vi "CAN_initialize3.vi"() -> (0 "Array 2":errorcluster[](array[cluster]), 1 "Array":refnum<class "sbCANopenBaseClass.lvclass">[](array[class]), 2 "Motor order":i32[](array[numeric])=[3, 6, 9, 12, 2, 7, 8, 13, 4, 5, 10, 11, 1, 14])   [LabVIEW 2024]
uses:
  <vilib>/addons/Maxon Motor/EPOS2 CANopen/CANopen/sbCANopenBaseClass.lvclass
  <vilib>/addons/Maxon Motor/EPOS2 CANopen/EPOS2 Support Files/Typedefs/EPOS2 Config Data Input Current.ctl
  <vilib>/addons/Maxon Motor/EPOS2 CANopen/EPOS2 Support Files/Typedefs/EPOS2 Velocity Units.ctl
  <vilib>/addons/Maxon Motor/EPOS2 CANopen/EPOS2 Support Files/Polymorphic SubVIs/Config/EPOS2 Current Mode Configure.vi
  <vilib>/addons/Maxon Motor/EPOS2 CANopen/EPOS2 Library.lvlib
  <vilib>/addons/Maxon Motor/EPOS2 CANopen/CANopen/CANopen IndCom Interface/sdCANopenIndCom.lvclass
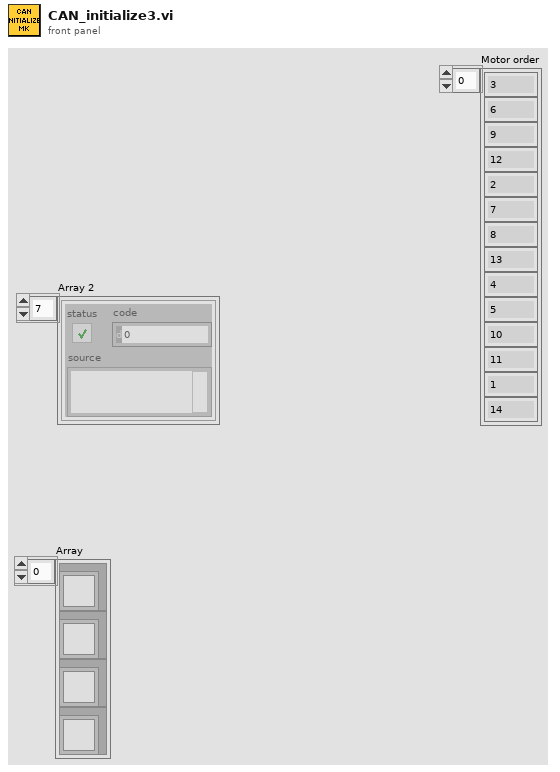
[diagram p1: front panel]
types:
  T1 = typedef "EPOS2 Library.lvlib/EPOS2 Config Data Input Current.ctl" = cluster{"Velocity Units":T2, "Max Velocity":i32}
  T2 = typedef "EPOS2 Library.lvlib/EPOS2 Velocity Units.ctl" = i8
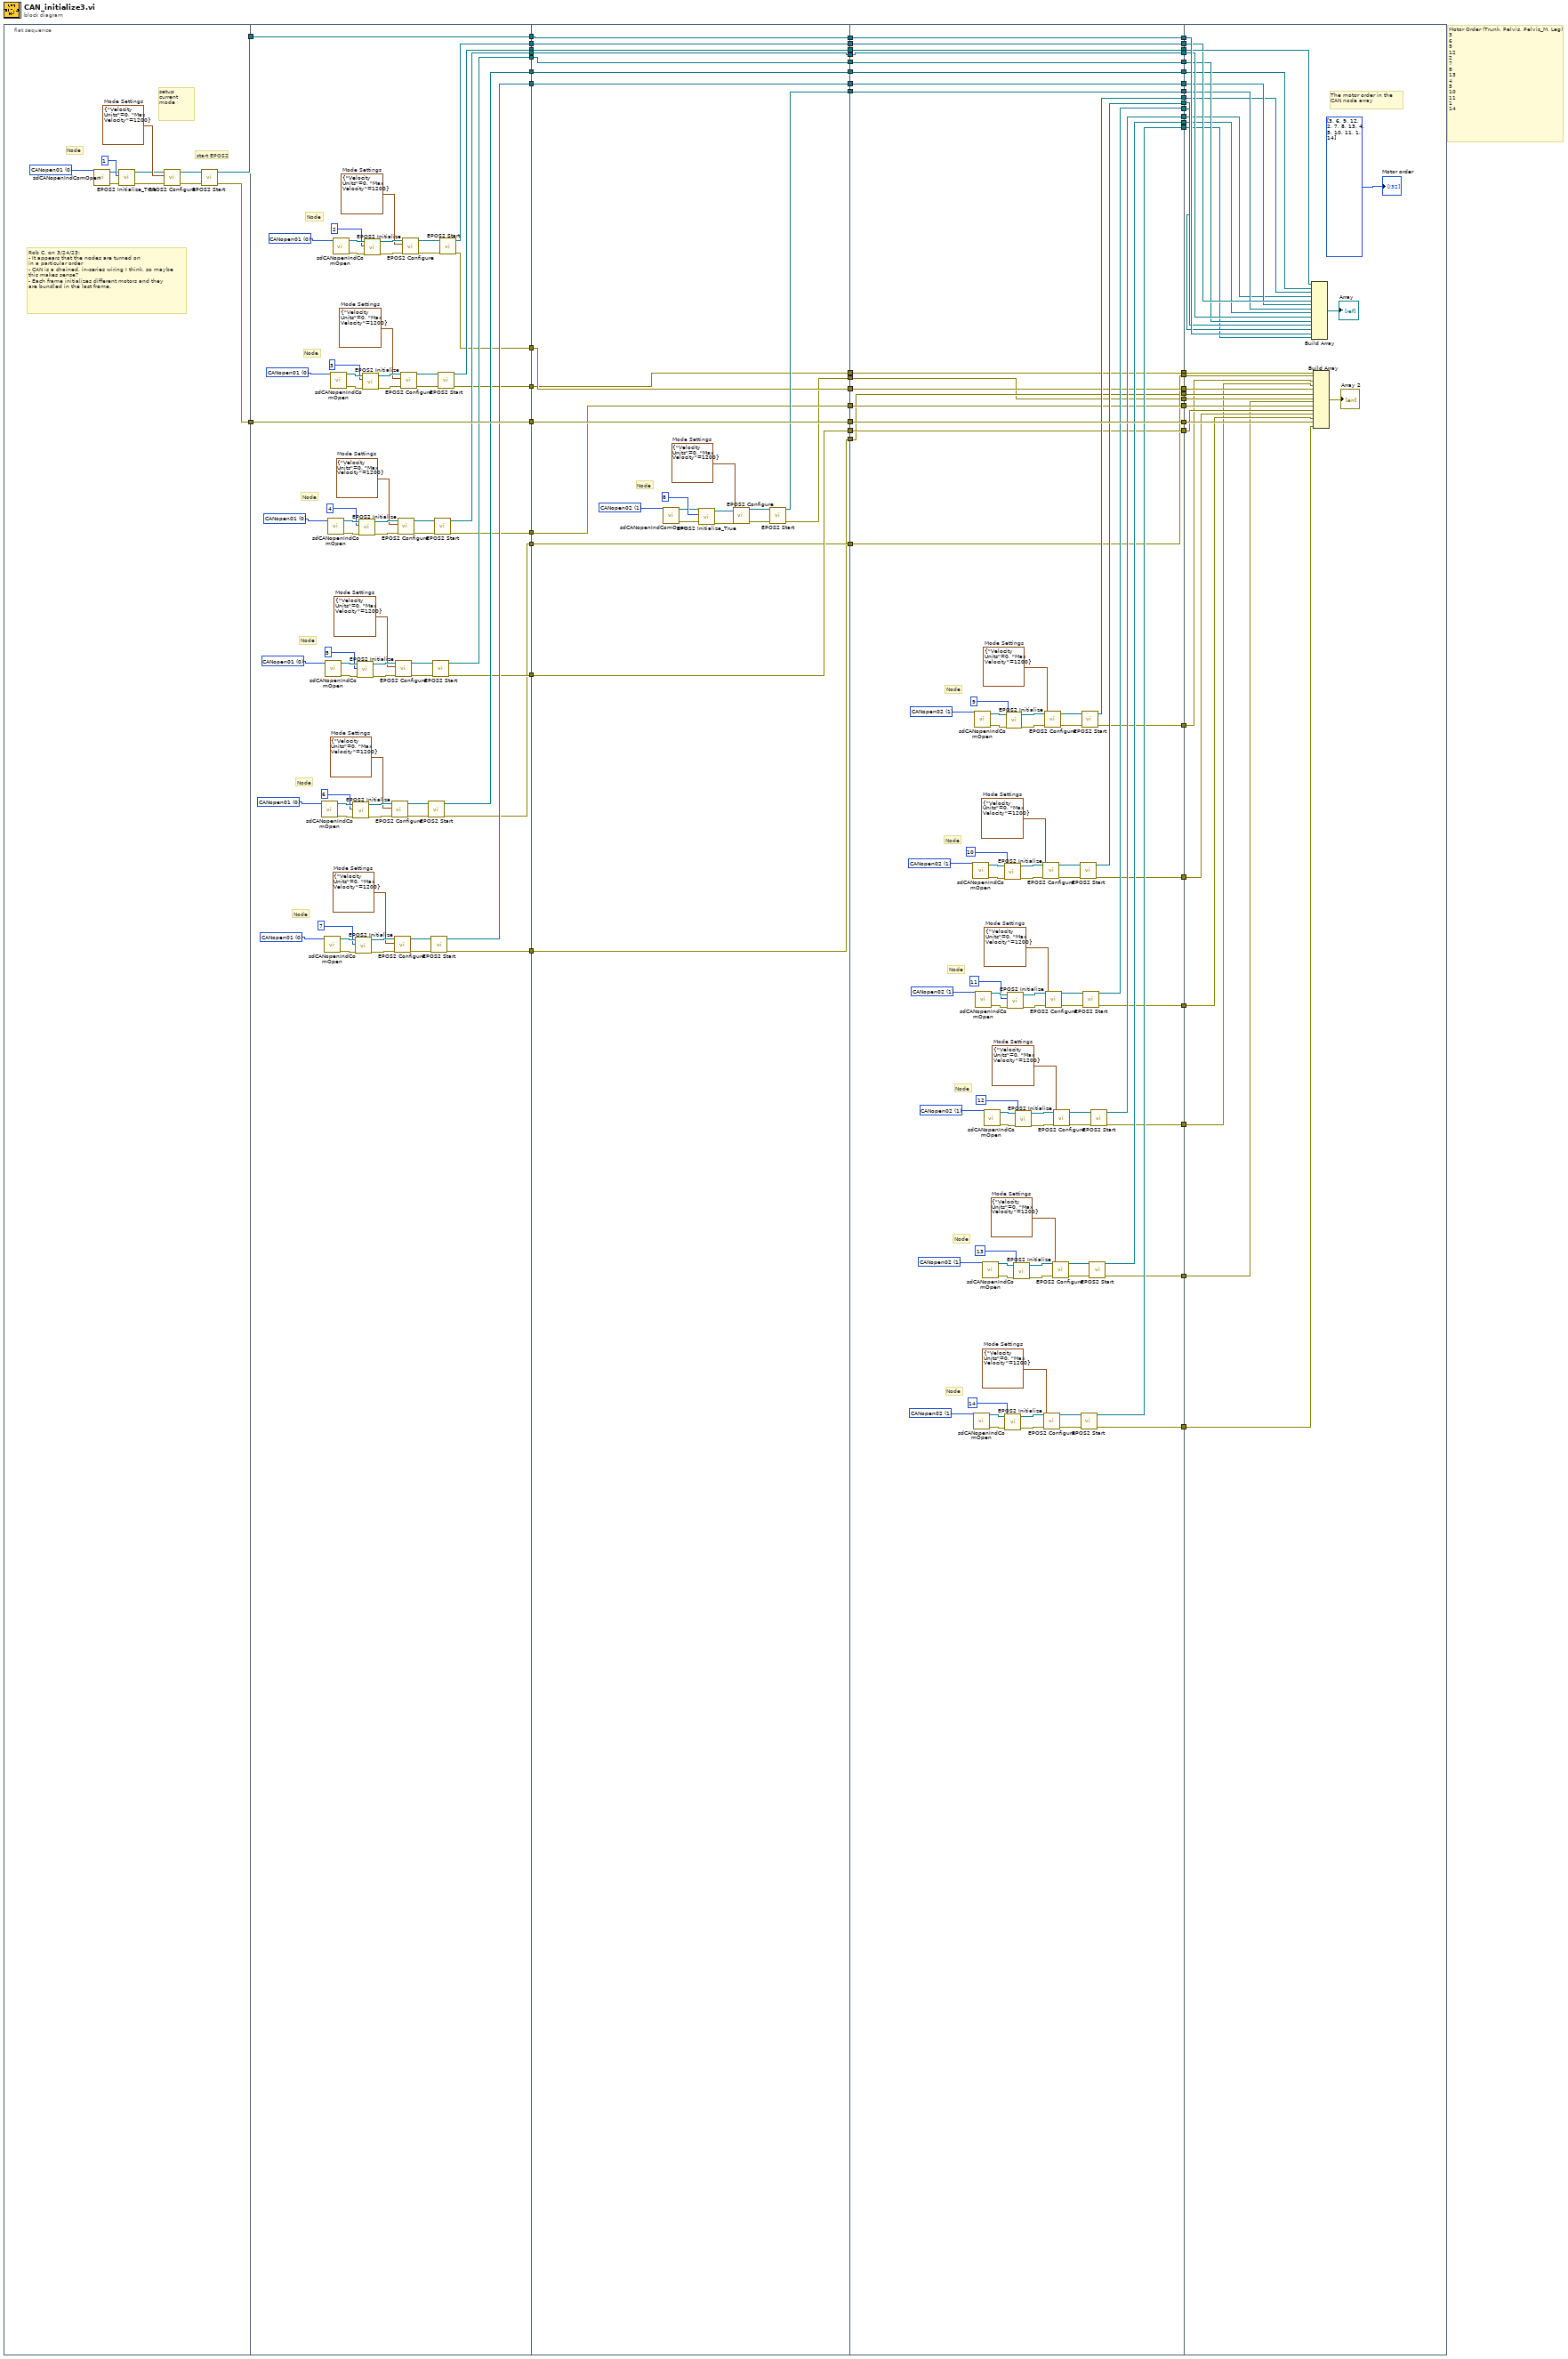
[diagram p0: block diagram]
diagram:
  # "Motor Order (Trunk, Pelvis, Pelvis_M, Leg)\n3\n6\n9\n12\n2\n7\n8\n13\n4\n5\n10\n11\n1\n14"
  n1 = flat-sequence {
    tunnel: [w62] -> w60
    tunnel: [w61] -> w56
    tunnel: w60 -> [w85]
    tunnel: [w85] -> w57
    tunnel: w56 -> [w84]
    tunnel: [w84] -> w53
    tunnel: [w83] -> w50
    tunnel: [w82] -> w49
    tunnel: [w81] -> w46
    tunnel: [w80] -> w43
    tunnel: [w79] -> w38
    tunnel: [w78] -> w35
    tunnel: [w77] -> w26
    tunnel: [w76] -> w21
    tunnel: [w75] -> w18
    tunnel: [w74] -> w15
    tunnel: [w73] -> w14
    tunnel: [w72] -> w10
    tunnel: [w155] -> w58
    tunnel: w57 -> [w155]
    tunnel: [w154] -> w54
    tunnel: w53 -> [w154]
    tunnel: [w153] -> w51
    tunnel: w50 -> [w153]
    tunnel: w49 -> [w152]
    tunnel: [w152] -> w47
    tunnel: w46 -> [w151]
    tunnel: [w151] -> w44
    tunnel: w43 -> [w150]
    tunnel: [w150] -> w41
    tunnel: [w149] -> w39
    tunnel: w38 -> [w149]
    tunnel: [w148] -> w36
    tunnel: w35 -> [w148]
    tunnel: [w147] -> w34
    tunnel: w26 -> [w146]
    tunnel: [w146] -> w24
    tunnel: [w145] -> w22
    tunnel: w21 -> [w145]
    tunnel: [w144] -> w19
    tunnel: w18 -> [w144]
    tunnel: [w143] -> w16
    tunnel: w15 -> [w143]
    tunnel: w14 -> [w142]
    tunnel: [w142] -> w12
    tunnel: [w141] -> w11
    tunnel: w10 -> [w141]
    tunnel: [w140] -> w8
    tunnel: [w192] -> w59
    tunnel: w58 -> [w192]
    tunnel: [w191] -> w55
    tunnel: w54 -> [w191]
    tunnel: [w190] -> w52
    tunnel: w51 -> [w190]
    tunnel: [w189] -> w48
    tunnel: w47 -> [w189]
    tunnel: [w188] -> w45
    tunnel: w44 -> [w188]
    tunnel: [w187] -> w42
    tunnel: w41 -> [w187]
    tunnel: [w186] -> w40
    tunnel: w39 -> [w186]
    tunnel: [w185] -> w37
    tunnel: w36 -> [w185]
    tunnel: w34 -> [w184]
    tunnel: [w184] -> w33
    tunnel: [w183] -> w32
    tunnel: [w182] -> w31
    tunnel: [w181] -> w30
    tunnel: [w180] -> w29
    tunnel: [w179] -> w28
    tunnel: [w178] -> w27
    tunnel: [w177] -> w25
    tunnel: w24 -> [w177]
    tunnel: [w176] -> w23
    tunnel: w22 -> [w176]
    tunnel: [w175] -> w20
    tunnel: w19 -> [w175]
    tunnel: [w174] -> w17
    tunnel: w16 -> [w174]
    tunnel: [w173] -> w13
    tunnel: w12 -> [w173]
    tunnel: w11 -> [w172]
    tunnel: [w172] -> w9
    tunnel: w8 -> [w171]
    tunnel: [w171] -> w7
    tunnel: [w170] -> w6
    tunnel: [w169] -> w5
    tunnel: [w168] -> w4
    tunnel: [w167] -> w3
    tunnel: [w166] -> w2
    tunnel: [w165] -> w1
    tunnel: w59 -> [w277]
    tunnel: w55 -> [w276]
    tunnel: w52 -> [w272]
    tunnel: w48 -> [w273]
    tunnel: w45 -> [w271]
    tunnel: w42 -> [w270]
    tunnel: w40 -> [w269]
    tunnel: w37 -> [w268]
    tunnel: w33 -> [w267]
    tunnel: w32 -> [w266]
    tunnel: w31 -> [w265]
    tunnel: w30 -> [w264]
    tunnel: w29 -> [w263]
    tunnel: w28 -> [w262]
    tunnel: w27 -> [w261]
    tunnel: w25 -> [w260]
    tunnel: w23 -> [w259]
    tunnel: w20 -> [w258]
    tunnel: w17 -> [w257]
    tunnel: w13 -> [w256]
    tunnel: w9 -> [w255]
    tunnel: w7 -> [w254]
    tunnel: w6 -> [w253]
    tunnel: w5 -> [w252]
    tunnel: w4 -> [w251]
    tunnel: w3 -> [w250]
    tunnel: w2 -> [w249]
    tunnel: w1 -> [w248]
    frame #0 {
      w70 = u32 0 items=["CANopen01", "CANopen02", "CANopen03", "CANopen04", "CANopen05", "CANopen06", "CANopen07", "CANopen08", "CANopen09", "CANopen10", "CANopen11", "CANopen12", "CANopen13", "CANopen14", "CANopen15", "CANopen16", "CANopen17", "CANopen18", "CANopen19", "CANopen20", "CANopen21", "CANopen22", "CANopen23", "CANopen24", "CANopen25", "CANopen26", "CANopen27", "CANopen28", "CANopen29", "CANopen30", "CANopen31", "CANopen32"] ("Interface Name")
      w71 = T1 {"Velocity Units"=0, "Max Velocity"=1200}  # Mode Settings
      # "Rob C. on 3/24/23:\n- It appears that the nodes are turned on\nin a particular order\n- CAN is a chained, in-series wiring I think, so maybe\nthis makes sense? \n- Each frame initializes different motors and they \nare bundled in the last frame."
      # "Node"
      # "start EPOS2"
      # "setup current mode"
      n2 = call <vilib>:"sdCANopenIndComOpen.vi"("Interface Name"=w70) -> ("error out"=w67:errorcluster, "SD CANopen Comm out"=w63:refnum<class "sbCANopenBaseClass.lvclass">)  [unwired: 9 in]
      n3 = call <vilib>:"EPOS2 Initialize_True.vi"("error in"=w67, "Node ID"=u8 1, "CAN Session In"=w63) -> ("error out"=w68:errorcluster, "CANopen Session Out"=w65:refnum<class "sbCANopenBaseClass.lvclass">)  [unwired: 7 in]
      n4 = call-poly <vilib>:"EPOS2 Configure.vi"("error in"=w68, "Mode Settings"=w71, "CANopen Session In"=w65) -> ("error out"=w66:errorcluster, "CANopen Session Out"=w64:refnum<class "sbCANopenBaseClass.lvclass">)  [unwired: 7 in]
      n5 = call <vilib>:"EPOS2 Start.vi"("error in"=w66, "CANopen Session In"=w64) -> ("error out"=w61:errorcluster, "CANopen Session Out"=w62:refnum<class "sbCANopenBaseClass.lvclass">)  [unwired: 8 in]
    }
    frame #1 {
      w89 = u32 0 items=["CANopen01", "CANopen02", "CANopen03", "CANopen04", "CANopen05", "CANopen06", "CANopen07", "CANopen08", "CANopen09", "CANopen10", "CANopen11", "CANopen12", "CANopen13", "CANopen14", "CANopen15", "CANopen16", "CANopen17", "CANopen18", "CANopen19", "CANopen20", "CANopen21", "CANopen22", "CANopen23", "CANopen24", "CANopen25", "CANopen26", "CANopen27", "CANopen28", "CANopen29", "CANopen30", "CANopen31", "CANopen32"] ("Interface Name")
      w90 = T1 {"Velocity Units"=0, "Max Velocity"=1200}  # Mode Settings
      w97 = u32 0 items=["CANopen01", "CANopen02", "CANopen03", "CANopen04", "CANopen05", "CANopen06", "CANopen07", "CANopen08", "CANopen09", "CANopen10", "CANopen11", "CANopen12", "CANopen13", "CANopen14", "CANopen15", "CANopen16", "CANopen17", "CANopen18", "CANopen19", "CANopen20", "CANopen21", "CANopen22", "CANopen23", "CANopen24", "CANopen25", "CANopen26", "CANopen27", "CANopen28", "CANopen29", "CANopen30", "CANopen31", "CANopen32"] ("Interface Name")
      w98 = T1 {"Velocity Units"=0, "Max Velocity"=1200}  # Mode Settings
      w109 = u32 0 items=["CANopen01", "CANopen02", "CANopen03", "CANopen04", "CANopen05", "CANopen06", "CANopen07", "CANopen08", "CANopen09", "CANopen10", "CANopen11", "CANopen12", "CANopen13", "CANopen14", "CANopen15", "CANopen16", "CANopen17", "CANopen18", "CANopen19", "CANopen20", "CANopen21", "CANopen22", "CANopen23", "CANopen24", "CANopen25", "CANopen26", "CANopen27", "CANopen28", "CANopen29", "CANopen30", "CANopen31", "CANopen32"] ("Interface Name")
      w110 = T1 {"Velocity Units"=0, "Max Velocity"=1200}  # Mode Settings
      w117 = u32 0 items=["CANopen01", "CANopen02", "CANopen03", "CANopen04", "CANopen05", "CANopen06", "CANopen07", "CANopen08", "CANopen09", "CANopen10", "CANopen11", "CANopen12", "CANopen13", "CANopen14", "CANopen15", "CANopen16", "CANopen17", "CANopen18", "CANopen19", "CANopen20", "CANopen21", "CANopen22", "CANopen23", "CANopen24", "CANopen25", "CANopen26", "CANopen27", "CANopen28", "CANopen29", "CANopen30", "CANopen31", "CANopen32"] ("Interface Name")
      w118 = T1 {"Velocity Units"=0, "Max Velocity"=1200}  # Mode Settings
      w125 = u32 0 items=["CANopen01", "CANopen02", "CANopen03", "CANopen04", "CANopen05", "CANopen06", "CANopen07", "CANopen08", "CANopen09", "CANopen10", "CANopen11", "CANopen12", "CANopen13", "CANopen14", "CANopen15", "CANopen16", "CANopen17", "CANopen18", "CANopen19", "CANopen20", "CANopen21", "CANopen22", "CANopen23", "CANopen24", "CANopen25", "CANopen26", "CANopen27", "CANopen28", "CANopen29", "CANopen30", "CANopen31", "CANopen32"] ("Interface Name")
      w126 = T1 {"Velocity Units"=0, "Max Velocity"=1200}  # Mode Settings
      w133 = u32 0 items=["CANopen01", "CANopen02", "CANopen03", "CANopen04", "CANopen05", "CANopen06", "CANopen07", "CANopen08", "CANopen09", "CANopen10", "CANopen11", "CANopen12", "CANopen13", "CANopen14", "CANopen15", "CANopen16", "CANopen17", "CANopen18", "CANopen19", "CANopen20", "CANopen21", "CANopen22", "CANopen23", "CANopen24", "CANopen25", "CANopen26", "CANopen27", "CANopen28", "CANopen29", "CANopen30", "CANopen31", "CANopen32"] ("Interface Name")
      w134 = T1 {"Velocity Units"=0, "Max Velocity"=1200}  # Mode Settings
      # "Node"
      # "Node"
      # "Node"
      # "Node"
      # "Node"
      # "Node"
      n6 = call <vilib>:"sdCANopenIndComOpen.vi"("Interface Name"=w97) -> ("error out"=w102:errorcluster, "SD CANopen Comm out"=w96:refnum<class "sbCANopenBaseClass.lvclass">)  [unwired: 9 in]
      n7 = call <vilib>:"sdCANopenIndComOpen.vi"("Interface Name"=w89) -> ("error out"=w94:errorcluster, "SD CANopen Comm out"=w88:refnum<class "sbCANopenBaseClass.lvclass">)  [unwired: 9 in]
      n8 = call <vilib>:"sdCANopenIndComOpen.vi"("Interface Name"=w109) -> ("error out"=w114:errorcluster, "SD CANopen Comm out"=w108:refnum<class "sbCANopenBaseClass.lvclass">)  [unwired: 9 in]
      n9 = call <vilib>:"sdCANopenIndComOpen.vi"("Interface Name"=w117) -> ("error out"=w122:errorcluster, "SD CANopen Comm out"=w116:refnum<class "sbCANopenBaseClass.lvclass">)  [unwired: 9 in]
      n10 = call <vilib>:"sdCANopenIndComOpen.vi"("Interface Name"=w125) -> ("error out"=w130:errorcluster, "SD CANopen Comm out"=w124:refnum<class "sbCANopenBaseClass.lvclass">)  [unwired: 9 in]
      n11 = call <vilib>:"sdCANopenIndComOpen.vi"("Interface Name"=w133) -> ("error out"=w138:errorcluster, "SD CANopen Comm out"=w132:refnum<class "sbCANopenBaseClass.lvclass">)  [unwired: 9 in]
      n12 = call <vilib>:"EPOS2 Initialize.vi"("error in"=w102, "Node ID"=u8 6, "CAN Session In"=w96) -> ("error out"=w103:errorcluster, "CANopen Session Out"=w100:refnum<class "sbCANopenBaseClass.lvclass">)  [unwired: 1 in, 6 out]
      n13 = call <vilib>:"EPOS2 Initialize.vi"("error in"=w94, "Node ID"=u8 7, "CAN Session In"=w88) -> ("error out"=w95:errorcluster, "CANopen Session Out"=w92:refnum<class "sbCANopenBaseClass.lvclass">)  [unwired: 1 in, 6 out]
      n14 = call <vilib>:"EPOS2 Initialize.vi"("error in"=w114, "Node ID"=u8 5, "CAN Session In"=w108) -> ("error out"=w115:errorcluster, "CANopen Session Out"=w112:refnum<class "sbCANopenBaseClass.lvclass">)  [unwired: 1 in, 6 out]
      n15 = call <vilib>:"EPOS2 Initialize.vi"("error in"=w122, "Node ID"=u8 4, "CAN Session In"=w116) -> ("error out"=w123:errorcluster, "CANopen Session Out"=w120:refnum<class "sbCANopenBaseClass.lvclass">)  [unwired: 1 in, 6 out]
      n16 = call <vilib>:"EPOS2 Initialize.vi"("error in"=w130, "Node ID"=u8 3, "CAN Session In"=w124) -> ("error out"=w131:errorcluster, "CANopen Session Out"=w128:refnum<class "sbCANopenBaseClass.lvclass">)  [unwired: 1 in, 6 out]
      n17 = call <vilib>:"EPOS2 Initialize.vi"("error in"=w138, "Node ID"=u8 2, "CAN Session In"=w132) -> ("error out"=w139:errorcluster, "CANopen Session Out"=w136:refnum<class "sbCANopenBaseClass.lvclass">)  [unwired: 1 in, 6 out]
      n18 = call-poly <vilib>:"EPOS2 Configure.vi"("error in"=w103, "Mode Settings"=w98, "CANopen Session In"=w100) -> ("error out"=w101:errorcluster, "CANopen Session Out"=w99:refnum<class "sbCANopenBaseClass.lvclass">)  [unwired: 7 in]
      n19 = call-poly <vilib>:"EPOS2 Configure.vi"("error in"=w95, "Mode Settings"=w90, "CANopen Session In"=w92) -> ("error out"=w93:errorcluster, "CANopen Session Out"=w91:refnum<class "sbCANopenBaseClass.lvclass">)  [unwired: 7 in]
      n20 = call-poly <vilib>:"EPOS2 Configure.vi"("error in"=w115, "Mode Settings"=w110, "CANopen Session In"=w112) -> ("error out"=w113:errorcluster, "CANopen Session Out"=w111:refnum<class "sbCANopenBaseClass.lvclass">)  [unwired: 7 in]
      n21 = call-poly <vilib>:"EPOS2 Configure.vi"("error in"=w123, "Mode Settings"=w118, "CANopen Session In"=w120) -> ("error out"=w121:errorcluster, "CANopen Session Out"=w119:refnum<class "sbCANopenBaseClass.lvclass">)  [unwired: 7 in]
      n22 = call-poly <vilib>:"EPOS2 Configure.vi"("error in"=w131, "Mode Settings"=w126, "CANopen Session In"=w128) -> ("error out"=w129:errorcluster, "CANopen Session Out"=w127:refnum<class "sbCANopenBaseClass.lvclass">)  [unwired: 7 in]
      n23 = call-poly <vilib>:"EPOS2 Configure.vi"("error in"=w139, "Mode Settings"=w134, "CANopen Session In"=w136) -> ("error out"=w137:errorcluster, "CANopen Session Out"=w135:refnum<class "sbCANopenBaseClass.lvclass">)  [unwired: 7 in]
      n24 = call <vilib>:"EPOS2 Start.vi"("error in"=w101, "CANopen Session In"=w99) -> ("error out"=w73:errorcluster, "CANopen Session Out"=w79:refnum<class "sbCANopenBaseClass.lvclass">)  [unwired: 8 in]
      n25 = call <vilib>:"EPOS2 Start.vi"("error in"=w93, "CANopen Session In"=w91) -> ("error out"=w72:errorcluster, "CANopen Session Out"=w78:refnum<class "sbCANopenBaseClass.lvclass">)  [unwired: 8 in]
      n26 = call <vilib>:"EPOS2 Start.vi"("error in"=w113, "CANopen Session In"=w111) -> ("error out"=w74:errorcluster, "CANopen Session Out"=w80:refnum<class "sbCANopenBaseClass.lvclass">)  [unwired: 8 in]
      n27 = call <vilib>:"EPOS2 Start.vi"("error in"=w121, "CANopen Session In"=w119) -> ("error out"=w75:errorcluster, "CANopen Session Out"=w81:refnum<class "sbCANopenBaseClass.lvclass">)  [unwired: 8 in]
      n28 = call <vilib>:"EPOS2 Start.vi"("error in"=w129, "CANopen Session In"=w127) -> ("error out"=w76:errorcluster, "CANopen Session Out"=w82:refnum<class "sbCANopenBaseClass.lvclass">)  [unwired: 8 in]
      n29 = call <vilib>:"EPOS2 Start.vi"("error in"=w137, "CANopen Session In"=w135) -> ("error out"=w77:errorcluster, "CANopen Session Out"=w83:refnum<class "sbCANopenBaseClass.lvclass">)  [unwired: 8 in]
    }
    frame #2 {
      w162 = u32 1 items=["CANopen01", "CANopen02", "CANopen03", "CANopen04", "CANopen05", "CANopen06", "CANopen07", "CANopen08", "CANopen09", "CANopen10", "CANopen11", "CANopen12", "CANopen13", "CANopen14", "CANopen15", "CANopen16", "CANopen17", "CANopen18", "CANopen19", "CANopen20", "CANopen21", "CANopen22", "CANopen23", "CANopen24", "CANopen25", "CANopen26", "CANopen27", "CANopen28", "CANopen29", "CANopen30", "CANopen31", "CANopen32"] ("Interface Name")
      w161 = T1 {"Velocity Units"=0, "Max Velocity"=1200}  # Mode Settings
      # "Node"
      n30 = call <vilib>:"sdCANopenIndComOpen.vi"("Interface Name"=w162) -> ("error out"=w157:errorcluster, "SD CANopen Comm out"=w159:refnum<class "sbCANopenBaseClass.lvclass">)  [unwired: 9 in]
      n31 = call <vilib>:"EPOS2 Initialize_True.vi"("error in"=w157, "Node ID"=u8 8, "CAN Session In"=w159) -> ("error out"=w156:errorcluster, "CANopen Session Out"=w158:refnum<class "sbCANopenBaseClass.lvclass">)  [unwired: 7 in]
      n32 = call-poly <vilib>:"EPOS2 Configure.vi"("error in"=w156, "Mode Settings"=w161, "CANopen Session In"=w158) -> ("error out"=w163:errorcluster, "CANopen Session Out"=w164:refnum<class "sbCANopenBaseClass.lvclass">)  [unwired: 7 in]
      n33 = call <vilib>:"EPOS2 Start.vi"("error in"=w163, "CANopen Session In"=w164) -> ("error out"=w140:errorcluster, "CANopen Session Out"=w147:refnum<class "sbCANopenBaseClass.lvclass">)  [unwired: 8 in]
    }
    frame #3 {
      w201 = u32 1 items=["CANopen01", "CANopen02", "CANopen03", "CANopen04", "CANopen05", "CANopen06", "CANopen07", "CANopen08", "CANopen09", "CANopen10", "CANopen11", "CANopen12", "CANopen13", "CANopen14", "CANopen15", "CANopen16", "CANopen17", "CANopen18", "CANopen19", "CANopen20", "CANopen21", "CANopen22", "CANopen23", "CANopen24", "CANopen25", "CANopen26", "CANopen27", "CANopen28", "CANopen29", "CANopen30", "CANopen31", "CANopen32"] ("Interface Name")
      w200 = T1 {"Velocity Units"=0, "Max Velocity"=1200}  # Mode Settings
      w198 = u32 1 items=["CANopen01", "CANopen02", "CANopen03", "CANopen04", "CANopen05", "CANopen06", "CANopen07", "CANopen08", "CANopen09", "CANopen10", "CANopen11", "CANopen12", "CANopen13", "CANopen14", "CANopen15", "CANopen16", "CANopen17", "CANopen18", "CANopen19", "CANopen20", "CANopen21", "CANopen22", "CANopen23", "CANopen24", "CANopen25", "CANopen26", "CANopen27", "CANopen28", "CANopen29", "CANopen30", "CANopen31", "CANopen32"] ("Interface Name")
      w197 = T1 {"Velocity Units"=0, "Max Velocity"=1200}  # Mode Settings
      w195 = u32 1 items=["CANopen01", "CANopen02", "CANopen03", "CANopen04", "CANopen05", "CANopen06", "CANopen07", "CANopen08", "CANopen09", "CANopen10", "CANopen11", "CANopen12", "CANopen13", "CANopen14", "CANopen15", "CANopen16", "CANopen17", "CANopen18", "CANopen19", "CANopen20", "CANopen21", "CANopen22", "CANopen23", "CANopen24", "CANopen25", "CANopen26", "CANopen27", "CANopen28", "CANopen29", "CANopen30", "CANopen31", "CANopen32"] ("Interface Name")
      w194 = T1 {"Velocity Units"=0, "Max Velocity"=1200}  # Mode Settings
      w228 = u32 1 items=["CANopen01", "CANopen02", "CANopen03", "CANopen04", "CANopen05", "CANopen06", "CANopen07", "CANopen08", "CANopen09", "CANopen10", "CANopen11", "CANopen12", "CANopen13", "CANopen14", "CANopen15", "CANopen16", "CANopen17", "CANopen18", "CANopen19", "CANopen20", "CANopen21", "CANopen22", "CANopen23", "CANopen24", "CANopen25", "CANopen26", "CANopen27", "CANopen28", "CANopen29", "CANopen30", "CANopen31", "CANopen32"] ("Interface Name")
      w227 = T1 {"Velocity Units"=0, "Max Velocity"=1200}  # Mode Settings
      w225 = u32 1 items=["CANopen01", "CANopen02", "CANopen03", "CANopen04", "CANopen05", "CANopen06", "CANopen07", "CANopen08", "CANopen09", "CANopen10", "CANopen11", "CANopen12", "CANopen13", "CANopen14", "CANopen15", "CANopen16", "CANopen17", "CANopen18", "CANopen19", "CANopen20", "CANopen21", "CANopen22", "CANopen23", "CANopen24", "CANopen25", "CANopen26", "CANopen27", "CANopen28", "CANopen29", "CANopen30", "CANopen31", "CANopen32"] ("Interface Name")
      w224 = T1 {"Velocity Units"=0, "Max Velocity"=1200}  # Mode Settings
      w222 = u32 1 items=["CANopen01", "CANopen02", "CANopen03", "CANopen04", "CANopen05", "CANopen06", "CANopen07", "CANopen08", "CANopen09", "CANopen10", "CANopen11", "CANopen12", "CANopen13", "CANopen14", "CANopen15", "CANopen16", "CANopen17", "CANopen18", "CANopen19", "CANopen20", "CANopen21", "CANopen22", "CANopen23", "CANopen24", "CANopen25", "CANopen26", "CANopen27", "CANopen28", "CANopen29", "CANopen30", "CANopen31", "CANopen32"] ("Interface Name")
      w221 = T1 {"Velocity Units"=0, "Max Velocity"=1200}  # Mode Settings
      # "Node"
      # "Node"
      # "Node"
      # "Node"
      # "Node"
      # "Node"
      n34 = call <vilib>:"sdCANopenIndComOpen.vi"("Interface Name"=w225) -> ("error out"=w239:errorcluster, "SD CANopen Comm out"=w235:refnum<class "sbCANopenBaseClass.lvclass">)  [unwired: 9 in]
      n35 = call <vilib>:"sdCANopenIndComOpen.vi"("Interface Name"=w201) -> ("error out"=w206:errorcluster, "SD CANopen Comm out"=w202:refnum<class "sbCANopenBaseClass.lvclass">)  [unwired: 9 in]
      n36 = call <vilib>:"sdCANopenIndComOpen.vi"("Interface Name"=w222) -> ("error out"=w245:errorcluster, "SD CANopen Comm out"=w241:refnum<class "sbCANopenBaseClass.lvclass">)  [unwired: 9 in]
      n37 = call <vilib>:"sdCANopenIndComOpen.vi"("Interface Name"=w228) -> ("error out"=w233:errorcluster, "SD CANopen Comm out"=w229:refnum<class "sbCANopenBaseClass.lvclass">)  [unwired: 9 in]
      n38 = call <vilib>:"sdCANopenIndComOpen.vi"("Interface Name"=w198) -> ("error out"=w212:errorcluster, "SD CANopen Comm out"=w208:refnum<class "sbCANopenBaseClass.lvclass">)  [unwired: 9 in]
      n39 = call <vilib>:"sdCANopenIndComOpen.vi"("Interface Name"=w195) -> ("error out"=w218:errorcluster, "SD CANopen Comm out"=w214:refnum<class "sbCANopenBaseClass.lvclass">)  [unwired: 9 in]
      n40 = call <vilib>:"EPOS2 Initialize.vi"("error in"=w239, "Node ID"=u8 10, "CAN Session In"=w235) -> ("error out"=w240:errorcluster, "CANopen Session Out"=w237:refnum<class "sbCANopenBaseClass.lvclass">)  [unwired: 1 in, 6 out]
      n41 = call <vilib>:"EPOS2 Initialize.vi"("error in"=w206, "Node ID"=u8 14, "CAN Session In"=w202) -> ("error out"=w207:errorcluster, "CANopen Session Out"=w204:refnum<class "sbCANopenBaseClass.lvclass">)  [unwired: 1 in, 6 out]
      n42 = call <vilib>:"EPOS2 Initialize.vi"("error in"=w245, "Node ID"=u8 9, "CAN Session In"=w241) -> ("error out"=w246:errorcluster, "CANopen Session Out"=w243:refnum<class "sbCANopenBaseClass.lvclass">)  [unwired: 1 in, 6 out]
      n43 = call <vilib>:"EPOS2 Initialize.vi"("error in"=w233, "Node ID"=u8 11, "CAN Session In"=w229) -> ("error out"=w234:errorcluster, "CANopen Session Out"=w231:refnum<class "sbCANopenBaseClass.lvclass">)  [unwired: 1 in, 6 out]
      n44 = call <vilib>:"EPOS2 Initialize.vi"("error in"=w212, "Node ID"=u8 13, "CAN Session In"=w208) -> ("error out"=w213:errorcluster, "CANopen Session Out"=w210:refnum<class "sbCANopenBaseClass.lvclass">)  [unwired: 1 in, 6 out]
      n45 = call <vilib>:"EPOS2 Initialize.vi"("error in"=w218, "Node ID"=u8 12, "CAN Session In"=w214) -> ("error out"=w219:errorcluster, "CANopen Session Out"=w216:refnum<class "sbCANopenBaseClass.lvclass">)  [unwired: 1 in, 6 out]
      n46 = call-poly <vilib>:"EPOS2 Configure.vi"("error in"=w240, "Mode Settings"=w224, "CANopen Session In"=w237) -> ("error out"=w238:errorcluster, "CANopen Session Out"=w236:refnum<class "sbCANopenBaseClass.lvclass">)  [unwired: 7 in]
      n47 = call-poly <vilib>:"EPOS2 Configure.vi"("error in"=w207, "Mode Settings"=w200, "CANopen Session In"=w204) -> ("error out"=w205:errorcluster, "CANopen Session Out"=w203:refnum<class "sbCANopenBaseClass.lvclass">)  [unwired: 7 in]
      n48 = call-poly <vilib>:"EPOS2 Configure.vi"("error in"=w246, "Mode Settings"=w221, "CANopen Session In"=w243) -> ("error out"=w244:errorcluster, "CANopen Session Out"=w242:refnum<class "sbCANopenBaseClass.lvclass">)  [unwired: 7 in]
      n49 = call-poly <vilib>:"EPOS2 Configure.vi"("error in"=w234, "Mode Settings"=w227, "CANopen Session In"=w231) -> ("error out"=w232:errorcluster, "CANopen Session Out"=w230:refnum<class "sbCANopenBaseClass.lvclass">)  [unwired: 7 in]
      n50 = call-poly <vilib>:"EPOS2 Configure.vi"("error in"=w213, "Mode Settings"=w197, "CANopen Session In"=w210) -> ("error out"=w211:errorcluster, "CANopen Session Out"=w209:refnum<class "sbCANopenBaseClass.lvclass">)  [unwired: 7 in]
      n51 = call-poly <vilib>:"EPOS2 Configure.vi"("error in"=w219, "Mode Settings"=w194, "CANopen Session In"=w216) -> ("error out"=w217:errorcluster, "CANopen Session Out"=w215:refnum<class "sbCANopenBaseClass.lvclass">)  [unwired: 7 in]
      n52 = call <vilib>:"EPOS2 Start.vi"("error in"=w238, "CANopen Session In"=w236) -> ("error out"=w169:errorcluster, "CANopen Session Out"=w182:refnum<class "sbCANopenBaseClass.lvclass">)  [unwired: 8 in]
      n53 = call <vilib>:"EPOS2 Start.vi"("error in"=w205, "CANopen Session In"=w203) -> ("error out"=w165:errorcluster, "CANopen Session Out"=w178:refnum<class "sbCANopenBaseClass.lvclass">)  [unwired: 8 in]
      n54 = call <vilib>:"EPOS2 Start.vi"("error in"=w244, "CANopen Session In"=w242) -> ("error out"=w170:errorcluster, "CANopen Session Out"=w183:refnum<class "sbCANopenBaseClass.lvclass">)  [unwired: 8 in]
      n55 = call <vilib>:"EPOS2 Start.vi"("error in"=w232, "CANopen Session In"=w230) -> ("error out"=w168:errorcluster, "CANopen Session Out"=w181:refnum<class "sbCANopenBaseClass.lvclass">)  [unwired: 8 in]
      n56 = call <vilib>:"EPOS2 Start.vi"("error in"=w211, "CANopen Session In"=w209) -> ("error out"=w166:errorcluster, "CANopen Session Out"=w179:refnum<class "sbCANopenBaseClass.lvclass">)  [unwired: 8 in]
      n57 = call <vilib>:"EPOS2 Start.vi"("error in"=w217, "CANopen Session In"=w215) -> ("error out"=w167:errorcluster, "CANopen Session Out"=w180:refnum<class "sbCANopenBaseClass.lvclass">)  [unwired: 8 in]
    }
    frame #4 {
      # "The motor order in the \nCAN node array"
      n58 = Build Array(w273, w269, w266, w263, w272, w268, w267, w262, w271, w270, w265, w264, w277, w261) -> (→"Array":refnum<class "sbCANopenBaseClass.lvclass">[])
      n59 = Build Array(w259, w256, w253, w250, w260, w255, w254, w249, w258, w257, w252, w251, w276, w248) -> (→"Array 2":errorcluster[])
      "Motor order" <- i32[] [3, 6, 9, 12, 2, 7, 8, 13, 4, 5, 10, 11, 1, 14]
    }
  }
